vi "loop daq.vi"(8 "error in (no error)":errorcluster, 11 "Template in":refnum<class "Template.lvclass">) -> ()   [LabVIEW 2020, in "Template.lvlib" / "Template.lvclass"]
doc: "Loop that hosts the Data Acquisition, Processing, Sending and Writing of the application.\nIf WriteData is defined as true, this module will write its own data as a separate file. If its defined as false, it will forward its data to the root actor, which in turn, will seek for an appropriate Data Writing actor to share this data."
uses:
  Template.lvclass
  Template.lvclass/Template.ctl
  accessors/Read Actor Events.vi
  accessors/Read Actor Notifiers.vi
  accessors/Read Actor Queues.vi
  accessors/Read This Actor Number.vi
  <vilib>/Utility/error.llb/Error Cluster From Error Code.vi
  interfaces/Error Interface/Error/Error.lvclass
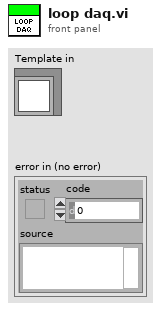
[diagram p1: front panel]
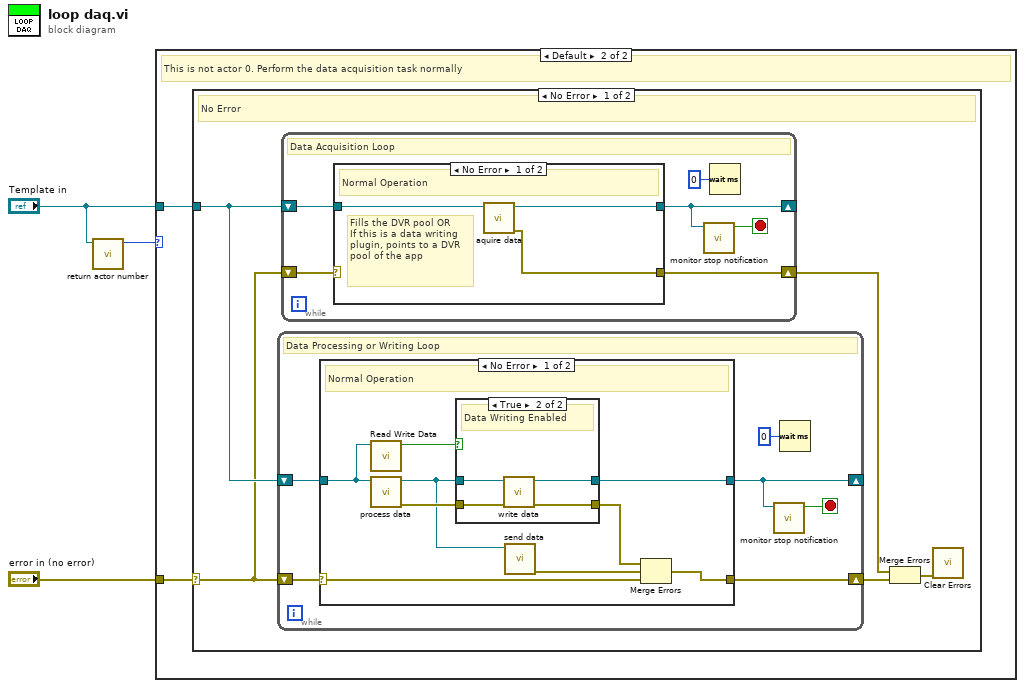
[diagram p0: block diagram]
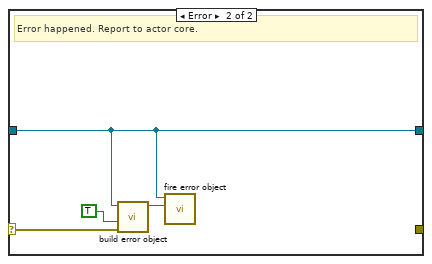
[diagram p4: hidden frame]
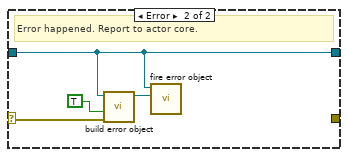
[diagram p5: hidden frame]
diagram:
  n1 = call "return actor number.vi"("Template in"="Template in") -> ("Actor number"=w1:u32)  [unwired: 10 in]
  n2 = case shown="Default" w1 {
    tunnel: "error in (no error)" -> [_ w5]
    tunnel: "Template in" -> [_ w4]
    frame 0 {
      # "This is actor 0.\nNo data acquisition should take place here"
    }
    frame Default {
      # "This is not actor 0. Perform the data acquisition task normally"
      n3 = case shown="No Error" w5 {
        selector: w5 -> [w9 _]
        tunnel: w4 -> [w10 _]
        frame No Error {
          # "No Error"
          n4 = while {
            shift-right: [w13] -> _
            shift-left: w10 -> [w16]
            shift-right: [w14] -> w8
            shift-left: w9 -> [w15]
            stop <- w12 stop-if-true
            # "Data Processing or Writing Loop"
            n5 = case shown="No Error" w15 {
              selector: w15 -> [w24 w33]
              tunnel: w16 -> [w18 w34]
              tunnel: [w25 w34] -> w13
              tunnel: [w22 _] -> w14
              frame No Error {
                # "Normal Operation"
                n6 = call "Read Write Data.vi"("Template in"=w18) -> ("WriteData"=w17:bool)  [unwired: 10 in]
                n7 = call-dynamic "process data.vi"("Template in"=w18) -> ("error out"=w23:errorcluster, "Template out"=w19:refnum<class "Template.lvclass">)  [unwired: 9 in]
                n8 = case shown="True" w17 {
                  tunnel: [w27 w31] -> w25
                  tunnel: w23 -> [w26 w30]
                  tunnel: [w26 w29] -> w20
                  tunnel: w19 -> [w27 w28]
                  frame False {
                    # "Data Writing Disabled"
                  }
                  frame True {
                    # "Data Writing Enabled"
                    n9 = call-dynamic "write data.vi"("error in (no error)"=w30, "Template in"=w28) -> ("error out"=w29:errorcluster, "Template out"=w31:refnum<class "Template.lvclass">)  [unwired: 8 in]
                  }
                }
                n10 = call "send data.vi"("Template in"=w19) -> ("error out"=w21:errorcluster)  [unwired: 10 in]
                n11 = Merge Errors(w20, w21, w24) -> (w22:errorcluster)
              }
              frame Error {
                # "Error happened. Report to actor core."
                n12 = call "build error object.vi"("Error to Process"=w33, "Report Error (F)"=TRUE, "Error Location"=w34) -> ("Error object"=w35:refnum<class>)  [unwired: 8 in]
                n13 = call "fire error object.vi"("Error in"=w35, "Template in"=w34) -> ()  [unwired: 10 in]
              }
            }
            n14 = call "monitor stop notification.vi"("Template in"=w13) -> ("Stop?"=w12:bool)  [unwired: 10 in]
            n15 = Wait (ms)(milliseconds to wait=u32 0) -> ()  [unwired: 1 out]
          }
          n16 = while {
            shift-right: [w38] -> _
            shift-left: w10 -> [w41]
            shift-right: [w39] -> w7
            shift-left: w9 -> [w40]
            stop <- w37 stop-if-true
            # "Data Acquisition Loop"
            n17 = case shown="No Error" w40 {
              selector: w40 -> [_ w46]
              tunnel: w41 -> [w44 w45]
              tunnel: [w43 w45] -> w38
              tunnel: [w42 _] -> w39
              frame No Error {
                # "Fills the DVR pool OR\nIf this is a data writing plugin, points to a DVR pool of the app"
                # "Normal Operation"
                n18 = call-dynamic "aquire data.vi"("Template in"=w44) -> ("error out"=w42:errorcluster, "Template out"=w43:refnum<class "Template.lvclass">)  [unwired: 9 in]
              }
              frame Error {
                # "Error happened. Report to actor core."
                n19 = call "build error object.vi"("Error to Process"=w46, "Report Error (F)"=TRUE, "Error Location"=w45) -> ("Error object"=w47:refnum<class>)  [unwired: 8 in]
                n20 = call "fire error object.vi"("Error in"=w47, "Template in"=w45) -> ()  [unwired: 10 in]
              }
            }
            n21 = call "monitor stop notification.vi"("Template in"=w38) -> ("Stop?"=w37:bool)  [unwired: 10 in]
            n22 = Wait (ms)(milliseconds to wait=u32 0) -> ()  [unwired: 1 out]
          }
          n23 = Merge Errors(w7, w8) -> (w6:errorcluster)
          n24 = call <vilib>:"Clear Errors.vi"("error in (no error)"=w6) -> ()  [unwired: 5 in, 2 out]
        }
        frame Error {
          # "Started in error. Do nothing."
        }
      }
    }
  }
